vi "Do.vi"(8 "error in (no error)":errorcluster, 10 "Actor in":refnum<class "Actor.lvclass">, 11 "Launch New Panel Msg":refnum<class "Launch New Panel Msg.lvclass">) -> (0 "error out":errorcluster, 2 "Actor out":refnum<class "Actor.lvclass">)   [LabVIEW 2015, in "Launch New Panel Msg.lvclass"]
doc: "(<B>Filename</B>: Actor Framework.lvlib:Message.lvclass:Do.vi)\n\nDefines what a message does when it is received by an actor. Generally, a message instructs an actor to invoke one of its methods. By default, this method does nothing. A child class must override it to define behavior. Create a child class by using the Actor Framework Message Maker dialog box."
uses:
  Launch New Panel Msg.lvclass
  <vilib>/ActorFramework/Actor/Actor.lvclass
  Panel Manager/Panel Manager Controller.lvclass
  Launch New Panel Msg.lvclass/Launch New Panel Msg.ctl
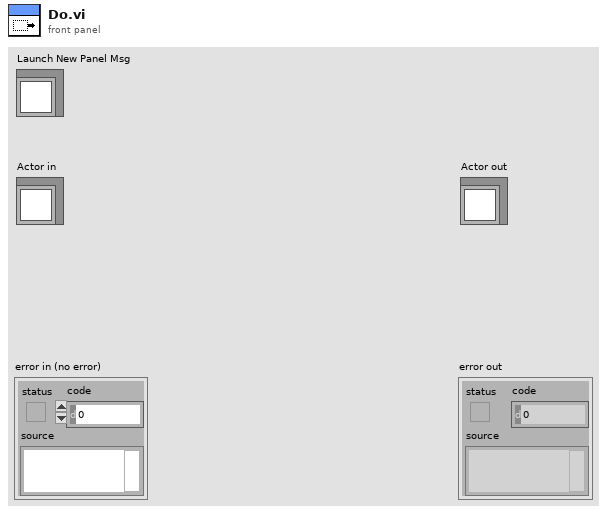
[diagram p1: front panel]
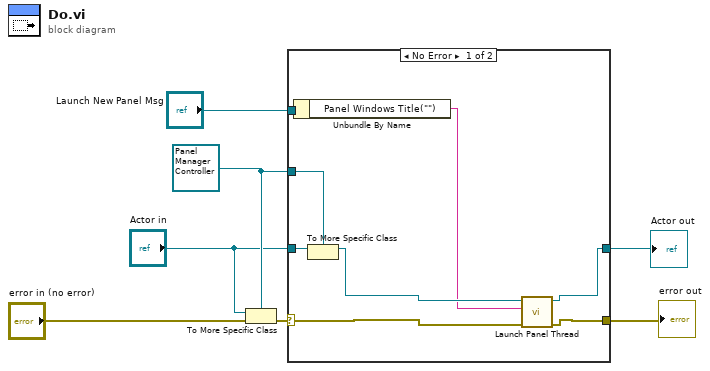
[diagram p0: block diagram]
diagram:
  w6 = refnum<class "Panel Manager Controller.lvclass"> refnum ("Panel Manager Controller.lvclass")
  n1 = To More Specific Class(target class=w6, reference="Actor in", error in="error in (no error)") -> (error out=w7:errorcluster)  [unwired: 1 out]
  n2 = case shown="No Error" w7 {
    selector: w7 -> [w10 w17]
    tunnel: [w9 w17] -> w2
    tunnel: [w11 w16] -> w4
    tunnel: "Actor in" -> [w15 w16]
    tunnel: w6 -> [w14 _]
    tunnel: "Launch New Panel Msg" -> [w13 _]
    frame No Error {
      n3 = Unbundle By Name(w13) -> ("Panel Windows Title(\"\")"=w8:string)
      n4 = To More Specific Class(target class=w14, reference=w15) -> (specific class reference=w12:refnum<class "Panel Manager Controller.lvclass">)  [unwired: 1 in, 1 out]
      n5 = call "Launch Panel Thread.vi"("error in (no error)"=w10, "Front Panel Window:Title(\"\")"=w8, "Panel Manager Controller.lvclass"=w12) -> ("error out"=w9:errorcluster, "Panel Manager Controller.lvclass out"=w11:refnum<class "Panel Manager Controller.lvclass">)  [unwired: 7 in]
    }
    frame Error {
      # "If type check fails, pass the original object out again."
    }
  }
  "error out" <- w2
  "Actor out" <- w4
